vi "Disabled.vi"(7 "Robot Mode":T2, 10 "Match Info":T1={"Autonomous Elapsed Seconds"=0.0, "TeleOp Elapsed Seconds"=0.0, "Disabled Elapsed Seconds"=0.0, "Visited Autonomous"=FALSE, "Visited TeleOp"=FALSE, "Visited Disabled"=FALSE, "Autonomous Settings"={"Autonomous Style"=enum."Independent", "VI Refnum"=refnum}}, 11 "Call Context":T3) -> ()   [LabVIEW 2017]
doc: "This VI is called each time a disabled packet is received from the DS. It is often used to prepare for the next robot mode, to calibrate sensors, etc."
uses:
  <vilib>/Rock Robotics/WPI/DriverStation/WPI_DriverStationDerivedRobotMode.ctl
  <vilib>/Rock Robotics/WPI/DriverStation/WPI_DriverStationRobotMode2.ctl
  <vilib>/Rock Robotics/WPI/DriverStation/WPI_DriverStationMatch Info.ctl
  CommandTypes/LiftCommands.ctl
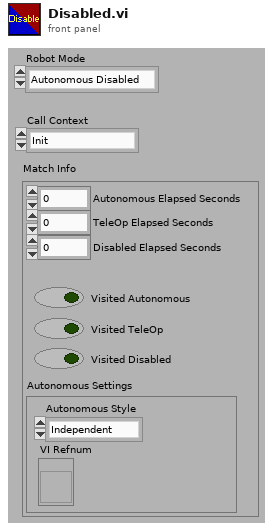
[diagram p1: front panel]
types:
  T1 = typedef "WPI_DriverStationMatch Info.ctl" = cluster{"Autonomous Elapsed Seconds":dbl, "TeleOp Elapsed Seconds":dbl, "Disabled Elapsed Seconds":dbl, "Visited Autonomous":bool, "Visited TeleOp":bool, "Visited Disabled":bool, "Autonomous Settings":cluster{"Autonomous Style":enum16{"Iterative", "Independent"}, "VI Refnum":refnum<vi>}}
  T2 = typedef "WPI_DriverStationRobotMode2.ctl" = enum16{"Autonomous Disabled", "Autonomous Enabled", "Teleop Disabled", "Teleop Enabled", "Disconnected", "Finish", "Test Disabled", "Test Enabled", "Emergency Stopped"}
  T3 = typedef "WPI_DriverStationDerivedRobotMode.ctl" = enum16{"Init", "Execute", "Stop"}
  T4 = typedef "LiftCommands.ctl" = enum16{"Do  Nothing", "Manuel", "Ground", "Home", "To Switch", "To Scale Low", "To Scale Medium", "To Scale High"}
  T5 = enum16{"Do Nothing", "Manuel", "Score", "Acquire"}
  T6 = enum16{"Center on Cube", "Manual", "Acquire Cube", "Drive Path"}
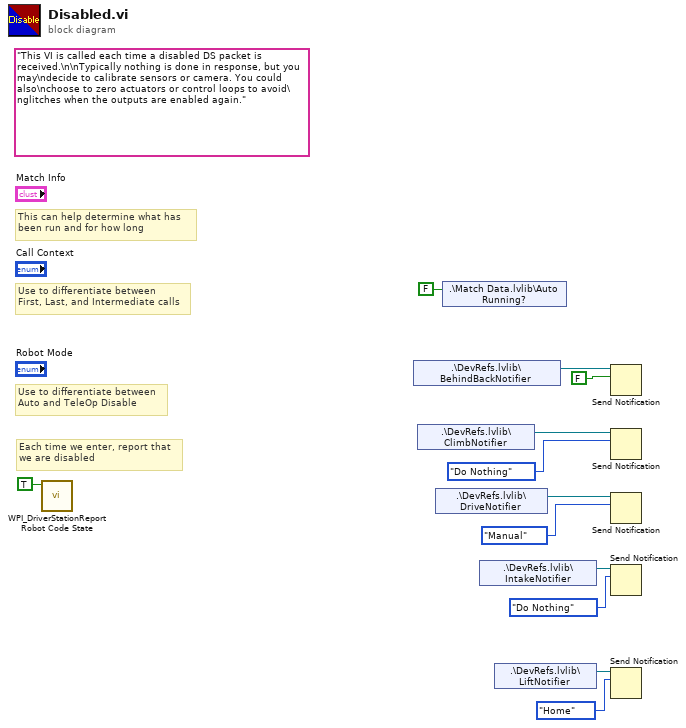
[diagram p0: block diagram]
diagram:
  (unwired) "This VI is called each time a disabled DS packet is received.\n\nTypically nothing is done in response, but you may\ndecide to calibrate sensors or camera. You could also\nchoose to zero actuators or control loops to avoid\nglitches when the outputs are enabled again."
  # "Each time we enter, report that\nwe are disabled"
  # "Use to differentiate between\nFirst, Last, and Intermediate calls"
  # "This can help determine what has\nbeen run and for how long"
  # "Use to differentiate between\nAuto and TeleOp Disable"
  n1 = call <vilib>:"WPI_DriverStationReport Robot Code State.vi"("Disabled"=TRUE ("Autonomous")) -> ()  [unwired: 10 in, 1 out]
  n2 = shared-variable ".\\DevRefs.lvlib\\BehindBackNotifier"() -> (w10:refnum<notifier>)  [unwired: 1 in, 1 out]
  n3 = shared-variable ".\\DevRefs.lvlib\\ClimbNotifier"() -> (w8:refnum<notifier>)  [unwired: 1 in, 1 out]
  n4 = shared-variable ".\\DevRefs.lvlib\\DriveNotifier"() -> (w6:refnum<notifier>)  [unwired: 1 in, 1 out]
  n5 = shared-variable ".\\Match Data.lvlib\\Auto Running?"(FALSE) -> ()  [unwired: 1 in, 1 out]
  n6 = shared-variable ".\\DevRefs.lvlib\\IntakeNotifier"() -> (w4:refnum<notifier>)  [unwired: 1 in, 1 out]
  n7 = shared-variable ".\\DevRefs.lvlib\\LiftNotifier"() -> (w2:refnum<notifier>)  [unwired: 1 in, 1 out]
  n8 = Send Notification(notification=FALSE, notifier=w10) -> ()  [unwired: 1 in, 2 out]
  n9 = Send Notification(notification=enum16{"Do Nothing", "Deploy", "Winch"}."Do Nothing", notifier=w8) -> ()  [unwired: 1 in, 2 out]
  n10 = Send Notification(notification=T6."Manual", notifier=w6) -> ()  [unwired: 1 in, 2 out]
  n11 = Send Notification(notification=T5."Do Nothing", notifier=w4) -> ()  [unwired: 1 in, 2 out]
  n12 = Send Notification(notification=LiftCommands."Home", notifier=w2) -> ()  [unwired: 1 in, 2 out]
